vi "Read frozen.vi"(8 "error in (no error)":errorcluster, 11 "PongBall in":refnum<class "PongBall.lvclass">) -> (0 "error out":errorcluster, 2 "frozen":bool, 3 "PongBall out":refnum<class "PongBall.lvclass">)   [LabVIEW 2019, in "RT_Game.lvlib" / "PongBall.lvclass"]
uses:
  PongBall.lvclass
  PongBall.lvclass/PongBall.ctl
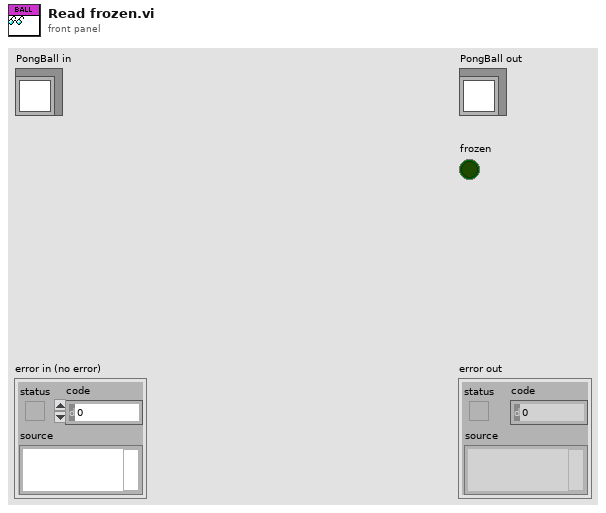
[diagram p1: front panel]
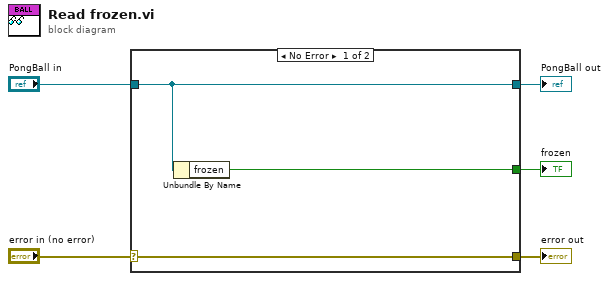
[diagram p0: block diagram]
diagram:
  n1 = case shown="No Error" "error in (no error)" {
    selector: "error in (no error)" -> [w8 w9]
    tunnel: [w8 w9] -> w4
    tunnel: [w7 w10] -> w2
    tunnel: "PongBall in" -> [w7 w10]
    tunnel: [w6 _] -> w1
    frame No Error {
      n2 = Unbundle By Name(w7) -> ("frozen"=w6:bool)
    }
    frame Error {
    }
  }
  "error out" <- w4
  "PongBall out" <- w2
  "frozen" <- w1
